vi "Main.vi"(8 "error in":errorcluster, 11 "TCP Server in":refnum<class "TCP Server.lvclass">) -> (0 "error out":errorcluster, 3 "TCP Server out":refnum<class "TCP Server.lvclass">)   [LabVIEW 2017, in "_TCP Server.lvlib" / "TCP Server.lvclass"]
doc: "The <b>Queued Message Handler</b> of the Worker that owns this VI."
uses:
  TCP Server.lvclass
  C:/SC/Source Code/VIPM/LabVIEW 20xx/vi.lib/addons/_Workers/Library/Classes/Worker/Worker.lvclass
  TCP Server.lvclass/TCP Server.ctl
  Initialization Data.ctl
  Response Cases.ctl
  <vilib>/addons/_Workers/Library/Case Label.ctl
  rql_Create Read Worker.ctl
  TCP Read/Initialization Data.ctl
  TCP Read/Response Cases.ctl
  <vilib>/addons/_Workers/Library/Classes/Message Queue/Message Queue.lvclass
  rqp_Start Listening.ctl
  TCP Listener/rqp_Listen for Connections.ctl
  rqp_Disconnect Clients.ctl
  rqp_Send String to Clients.ctl
  TCP Client Data.ctl
  <vilib>/addons/_Workers/Library/Classes/Message/Priority.ctl
  rsp_Connection Notify.ctl
  <vilib>/Utility/error.llb/Error Cluster From Error Code.vi
  <vilib>/addons/_Workers/Library/Classes/Worker/Worker.lvclass
  <vilib>/ErrorRing/Error Ring.xnode
  TCP Listener/TCP Listener.lvclass
  <vilib>/addons/_Workers/Library/Classes/Message/Message.lvclass
  TCP Read/TCP Read.lvclass
  <vilib>/addons/_Workers/Library/Workers.lvlib
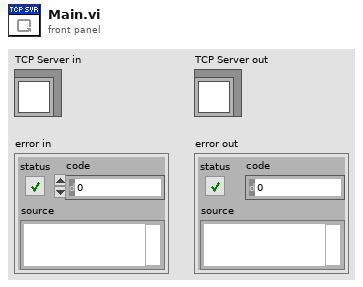
[diagram p1: front panel]
types:
  T1 = typedef "_TCP Server.lvlib/TCP Server.lvclass/Initialization Data.ctl" = cluster{"Response Cases":T2}
  T2 = typedef "_TCP Server.lvlib/TCP Server.lvclass/Response Cases.ctl" = cluster{"Incoming Data":T3, "Connection Notify":T3}
  T3 = typedef "Workers.lvlib/Case Label.ctl" = string
  T4 = typedef "_TCP Server.lvlib/TCP Read.lvclass/Initialization Data.ctl" = cluster{"Response Cases":T5, "Connection ID":refnum<k5>, "Forwarding Queue":refnum<class "Message Queue.lvclass">, "Forwarding Case":T3, "Client Name":string}
  T5 = typedef "_TCP Server.lvlib/TCP Read.lvclass/Response Cases.ctl" = cluster{"Connection Lost":T3}
  T6 = typedef "_TCP Server.lvlib/TCP Server.lvclass/rql_Create Read Worker.ctl" = cluster{"Connection ID":refnum<k5>, "Client Name":string}
  T7 = typedef "_TCP Server.lvlib/TCP Listener.lvclass/rqp_Listen for Connections.ctl" = cluster{"Server Name":string, "Server IP Address":u32, "Server Port":u16}
  T8 = typedef "_TCP Server.lvlib/TCP Server.lvclass/rqp_Start Listening.ctl" = cluster{"Server Name":string, "Server IP Address":string, "Server Port":u16}
  T9 = typedef "_TCP Server.lvlib/TCP Server.lvclass/rqp_Disconnect Clients.ctl" = cluster{"TCP Client Names":string[]}
  T10 = typedef "_TCP Server.lvlib/TCP Server.lvclass/rqp_Send String to Clients.ctl" = cluster{"TCP Client Names":string[], "String to Send":string}
  T11 = typedef "_TCP Server.lvlib/TCP Server.lvclass/rsp_Connection Notify.ctl" = cluster{"Client Name":string, "IP Address":string, "Connected?":bool}
  T12 = typedef "Workers.lvlib/Message.lvclass/Priority.ctl" = enum16{"Low", "Normal", "High"}
  T13 = typedef "_TCP Server.lvlib/TCP Server.lvclass/TCP Client Data.ctl" = cluster{"Connection ID":refnum<k5>, "Client Name":string, "IP Address":string}
  T14 = typedef "_TCP Server.lvlib/TCP Listener.lvclass/rsp_Add Listener.ctl" = cluster{"listener ID":refnum<k5>}
  T15 = typedef "_TCP Server.lvlib/TCP Listener.lvclass/rsp_New Connection.ctl" = cluster{"Connection ID":refnum<k5>, "Client Name":string, "IP Address":string}
  T16 = typedef "_TCP Server.lvlib/TCP Read.lvclass/rsp_Connection Lost.ctl" = cluster{"Connection ID":refnum<k5>, "TCP Read Queue":refnum<class "Message Queue.lvclass">}
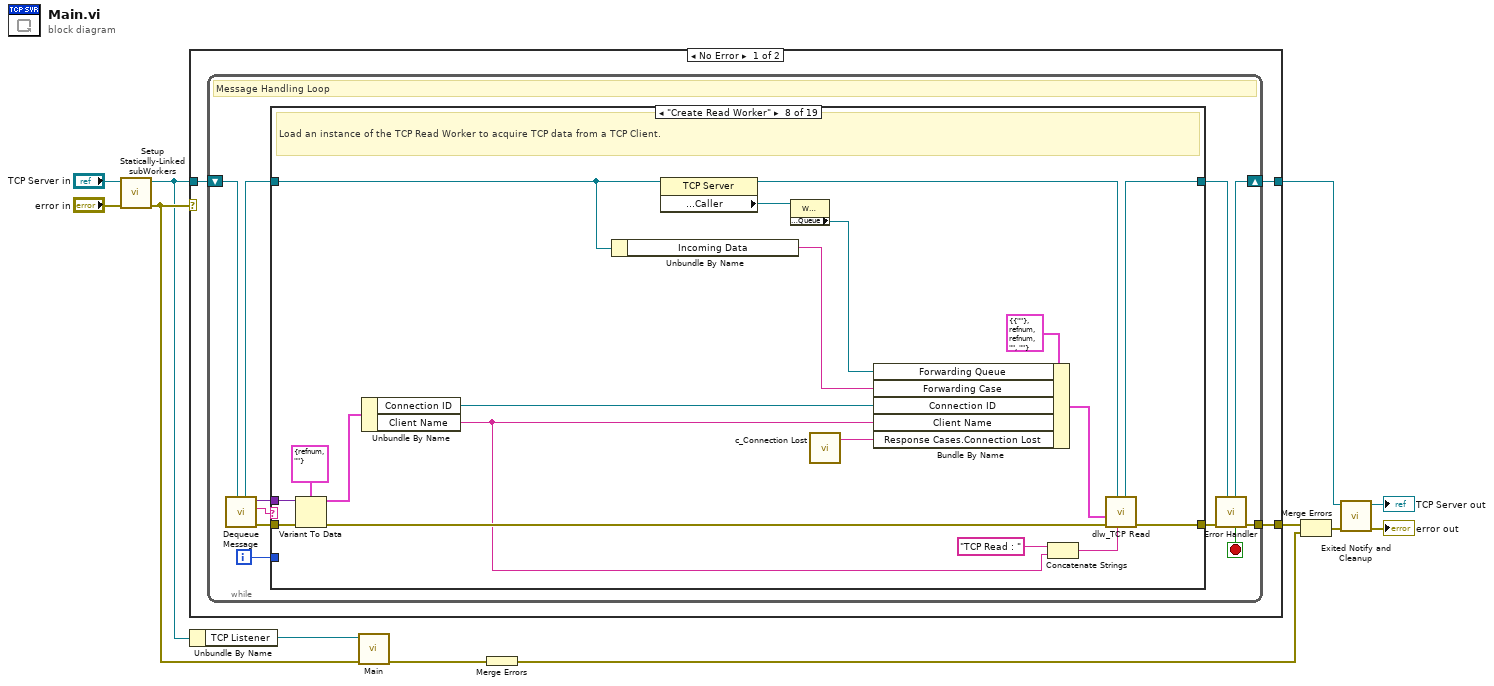
[diagram p0: block diagram]
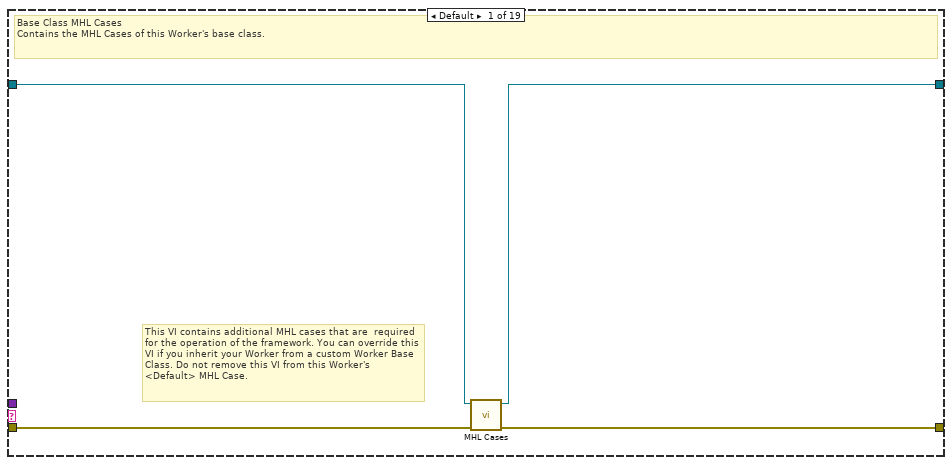
[diagram p2: hidden frame]
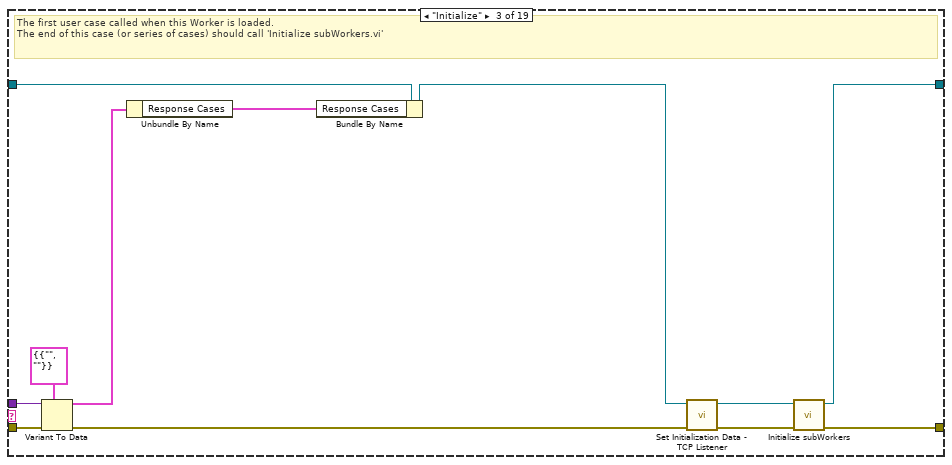
[diagram p4: hidden frame]
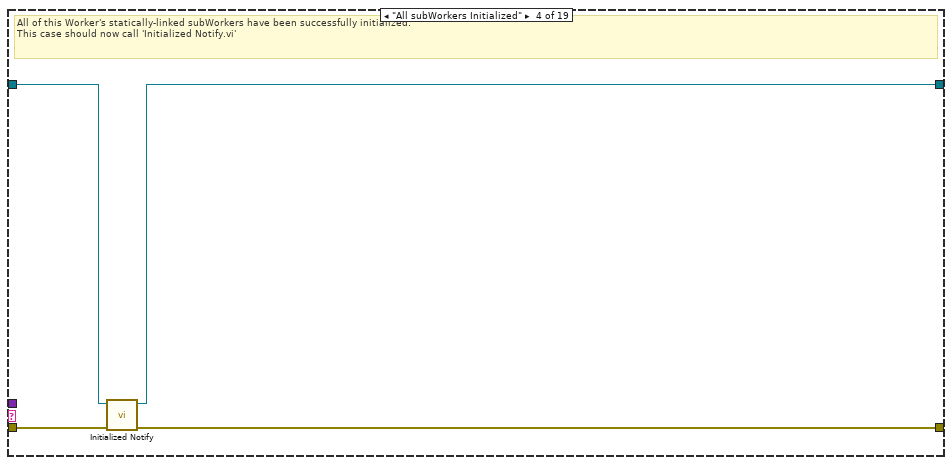
[diagram p5: hidden frame]
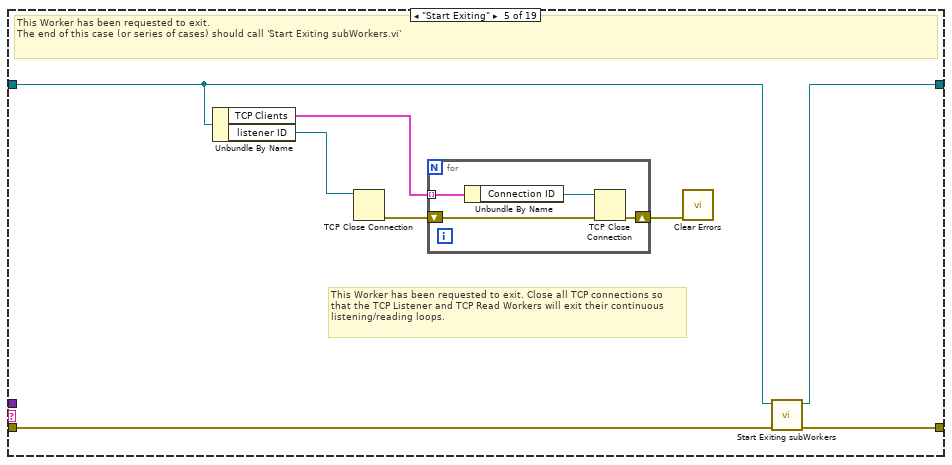
[diagram p6: hidden frame]
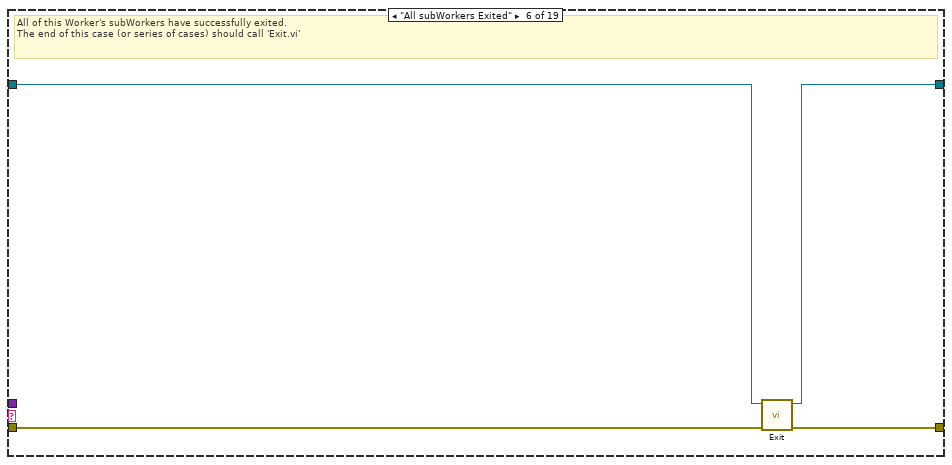
[diagram p7: hidden frame]
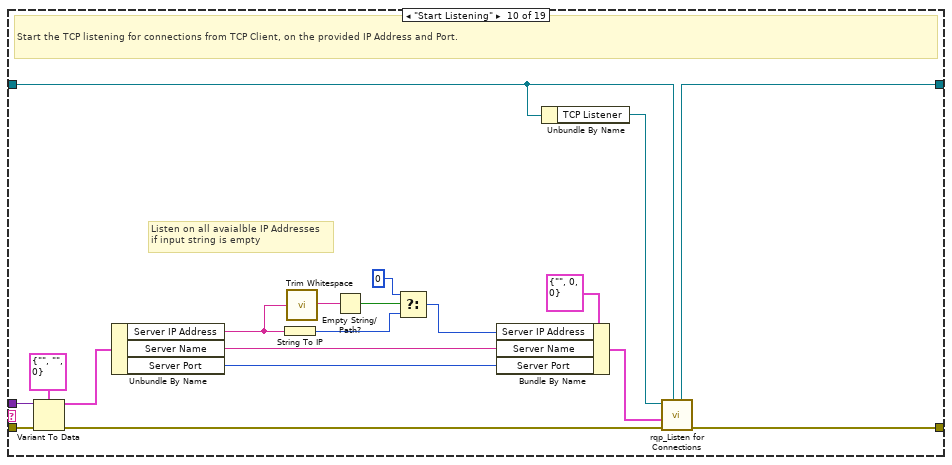
[diagram p10: hidden frame]
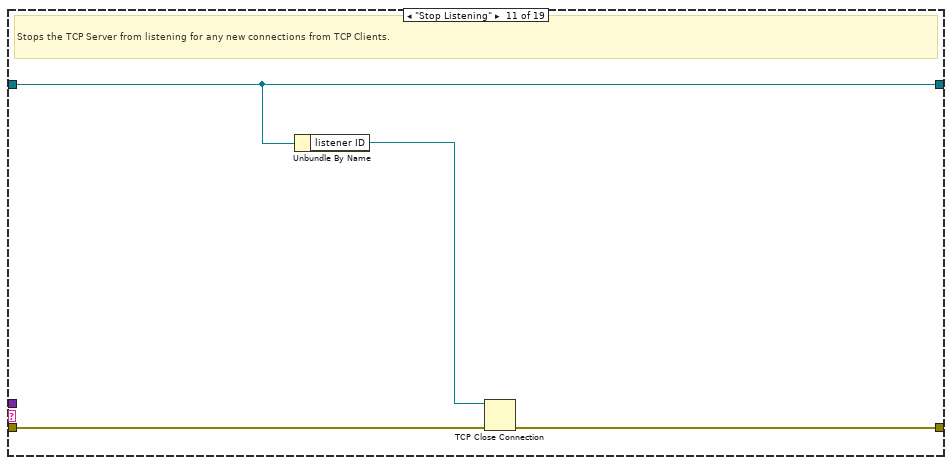
[diagram p11: hidden frame]
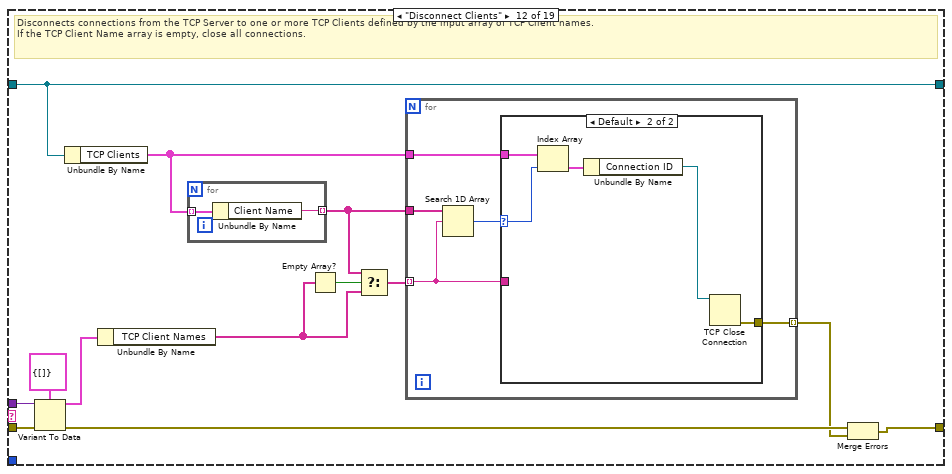
[diagram p12: hidden frame]
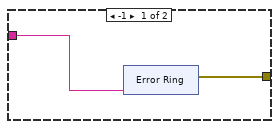
[diagram p13: hidden frame]
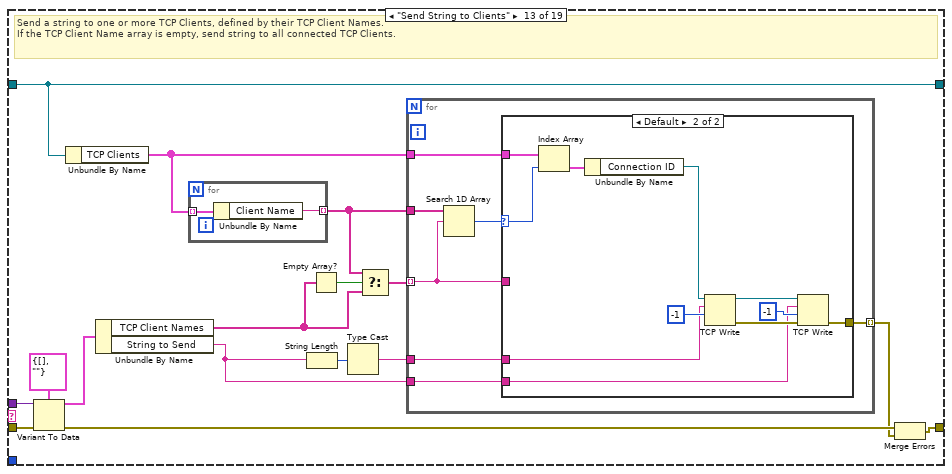
[diagram p14: hidden frame]
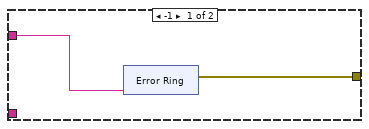
[diagram p15: hidden frame]
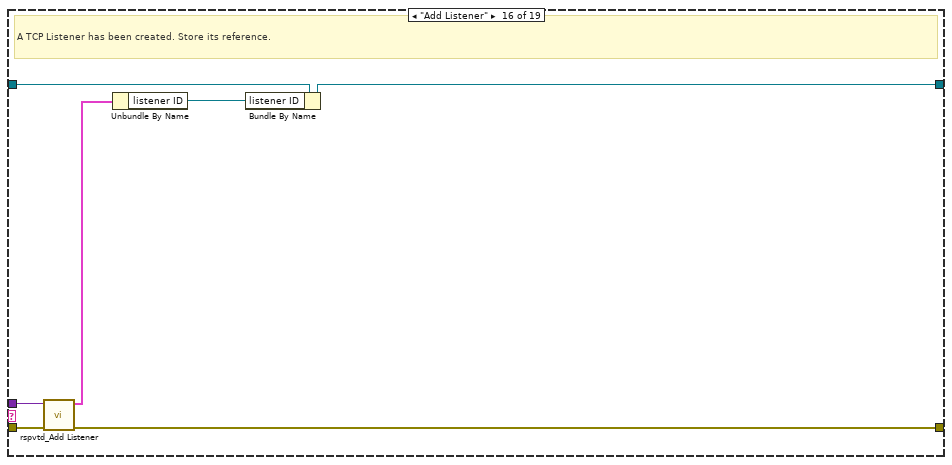
[diagram p18: hidden frame]
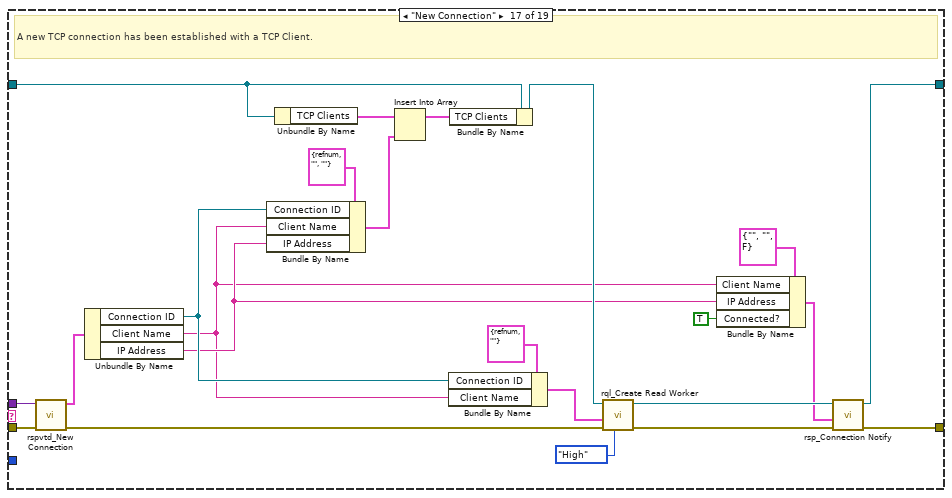
[diagram p19: hidden frame]
diagram:
  n1 = call "Setup Statically-Linked subWorkers.vi"("error in"="error in", "TCP Server in"="TCP Server in") -> ("error out"=w6:errorcluster, "TCP Server out"=w4:refnum<class "TCP Server.lvclass">)  [unwired: 8 in]
  n2 = case shown="No Error" w6 {
    tunnel: w4 -> [w13 w273]
    tunnel: [w15 w274] -> w11
    tunnel: [w14 w272] -> w12
    selector: w6 -> [_ w275]
    frame No Error {
      n3 = while {
        shift-right: [w24] -> w14
        shift-left: w13 -> [w26]
        tunnel: [w25] -> w15
        i -> [w17]
        stop <- w18 stop-if-true
        # "Message Handling Loop"
        n4 = call-dynamic "Dequeue Message.vi"("Worker"=w26) -> ("error out"=w23:errorcluster, "Case out"=w19:string, "Data out"=w16:variant, "Worker out"=w21:refnum<class "TCP Server.lvclass">)  [unwired: 6 in, 1 out]
        n5 = case "Worker MHL Case Structure (DO NOT CHANGE LABEL NAME)" shown="\"Create Read Worker\"" w19 {
          tunnel: w23 -> [w30 w31 w42 w48 w54 w64 w66 w85 w87 w106 w110 w123 w160 w191 w193 w200 w223 w225 w242]
          tunnel: [w29 w31 w44 w47 w56 w63 w66 w80 w87 w101 w109 w114 w149 w191 w193 w198 w208 w225 w235] -> w22
          tunnel: w21 -> [w28 w32 w41 w46 w53 w62 w65 w76 w86 w99 w108 w118 w153 w190 w192 w199 w218 w224 w238]
          tunnel: [w27 w32 w43 w45 w55 w61 w65 w79 w86 w100 w108 w118 w153 w190 w192 w195 w206 w224 w233] -> w20
          tunnel: w17 -> [_ _ _ _ _ _ _ _ _ _ _ _ _ _ _ _ _ _ _]
          tunnel: w16 -> [_ _ w39 _ _ _ _ w82 _ w104 _ w120 w157 _ _ w197 w222 _ w240]
          frame Default {
            # "This VI contains additional MHL cases that are  required for the operation of the framework. You can override this VI if you inherit your Worker from a custom Worker Base Class. Do not remove this VI from this Worker's <Default> MHL Case."
            # "Base Class MHL Cases\nContains the MHL Cases of this Worker's base class."
            n6 = call-dynamic "MHL Cases.vi"("error in"=w30, "Worker in"=w28) -> ("error out"=w29:errorcluster, "Worker out"=w27:refnum<class "TCP Server.lvclass">)  [unwired: 8 in]
          }
          frame "------------ FRAMEWORK CASES -----------" {
            # "Start of Workers Framework Cases"
          }
          frame "Initialize" {
            # "The first user case called when this Worker is loaded.\nThe end of this case (or series of cases) should call 'Initialize subWorkers.vi'"
            n7 = Variant To Data(error in=w42, type=T1 {"Response Cases"={"Incoming Data"="", "Connection Notify"=""}} ("Cluster"), Variant=w39) -> (data=w38:T1, error out=w40:errorcluster)
            n8 = Unbundle By Name(w38) -> ("Response Cases"=w37:T2)
            n9 = Bundle By Name(cluster=w41, "Response Cases"=w37) -> (w33:refnum<class "TCP Server.lvclass">)
            n10 = call "Set Initialization Data - TCP Listener.vi"("error in"=w40, "TCP Server in"=w33) -> ("error out"=w35:errorcluster, "TCP Server out"=w34:refnum<class "TCP Server.lvclass">)  [unwired: 8 in]
            n11 = call-dynamic "Initialize subWorkers.vi"("error in"=w35, "Worker"=w34) -> ("error out"=w44:errorcluster, "dup Worker out"=w43:refnum<class "TCP Server.lvclass">)  [unwired: 8 in]
          }
          frame "All subWorkers Initialized" {
            # "All of this Worker's statically-linked subWorkers have been successfully initialized.\nThis case should now call 'Initialized Notify.vi'"
            n12 = call-dynamic "Initialized Notify.vi"("error in"=w48, "Worker"=w46) -> ("error out"=w47:errorcluster, "dup Worker out"=w45:refnum<class "TCP Server.lvclass">)  [unwired: 8 in]
          }
          frame "Start Exiting" {
            # "This Worker has been requested to exit. Close all TCP connections so that the TCP Listener and TCP Read Workers will exit their continuous listening/reading loops."
            # "This Worker has been requested to exit. \nThe end of this case (or series of cases) should call 'Start Exiting subWorkers.vi'"
            n13 = Unbundle By Name(w53) -> ("TCP Clients"=w50:T13[], "listener ID"=w51:refnum<k5>)
            n14 = TCP Close Connection(connection ID=w51) -> (error out=w52:errorcluster)  [unwired: 2 in, 1 out]
            n15 = for {
              shift-right: [w59] -> w49
              shift-left: w52 -> [w60]
              tunnel: w50 -> [w58] mode=indexing
              n16 = Unbundle By Name(w58) -> ("Connection ID"=w57:refnum<k5>)
              n17 = TCP Close Connection(connection ID=w57, error in (no error)=w60) -> (error out=w59:errorcluster)  [unwired: 1 in, 1 out]
            }
            n18 = call <vilib>:"Clear Errors.vi"("error in (no error)"=w49) -> ()  [unwired: 5 in, 2 out]
            n19 = call-dynamic "Start Exiting subWorkers.vi"("error_in"=w54, "Worker"=w53) -> ("error out"=w56:errorcluster, "dup Worker out"=w55:refnum<class "TCP Server.lvclass">)  [unwired: 8 in]
          }
          frame "All subWorkers Exited" {
            # "All of this Worker's subWorkers have successfully exited. \nThe end of this case (or series of cases) should call 'Exit.vi'"
            n20 = call-dynamic "Exit.vi"("error_in"=w64, "Worker"=w62) -> ("error out"=w63:errorcluster, "dup Worker out"=w61:refnum<class "TCP Server.lvclass">)  [unwired: 8 in]
          }
          frame "------------- LOCAL API CASES -------------" {
            # "Start of Workers Local API Cases"
          }
          frame "Create Read Worker" {
            # "Load an instance of the TCP Read Worker to acquire TCP data from a TCP Client."
            n21 = Variant To Data(error in=w85, type=T6 {"Connection ID"=refnum, "Client Name"=""} ("Data"), Variant=w82) -> (data=w81:T6, error out=w84:errorcluster)
            n22 = Unbundle By Name(w81) -> ("Connection ID"=w72:refnum<k5>, "Client Name"=w70:string)
            n23 = Unbundle By Name(w76) -> ("Incoming Data"=w75:T3)
            n24 = property class="TCP Server"(reference=w76) -> (reference out=w74:refnum<class "TCP Server.lvclass">, "Accessors:Read:Public API:Caller"=w73:refnum<class "Worker.lvclass">)  [unwired: 1 in, 1 out]
            n25 = property class="Worker.lvclass"(reference=w73) -> ("Accessors:Read:Public API:Queue"=w67:refnum<class "Message Queue.lvclass">)  [unwired: 1 in, 2 out]
            n26 = call "c_Connection Lost.vi"() -> ("Case Label"=w68:T3)  [unwired: 1 in]
            n27 = Bundle By Name(cluster=T4 {"Response Cases"={"Connection Lost"=""}, "Connection ID"=refnum, "Forwarding Queue"=refnum, "Forwarding Case"="", "Client Name"=""} ("Initialization Data"), "Forwarding Queue"=w67, "Forwarding Case"=w75, "Connection ID"=w72, "Client Name"=w70, "Response Cases.Connection Lost"=w68) -> (w77:T4)
            n28 = Concatenate Strings("TCP Read : " ("Worker Alias"), w70) -> (w69:string)
            n29 = call "dlw_TCP Read.vi"("Worker Alias"=w69, "Caller in"=w74, "error in"=w84, "Initialization Data"=w77) -> ("error out"=w80:errorcluster, "dup Caller out"=w79:refnum<class "TCP Server.lvclass">)  [unwired: 5 in, 1 out]
          }
          frame "------------- PUBLIC API CASES -------------" {
            # "Start of Workers Public API Cases"
          }
          frame "Start Listening" {
            # "Listen on all avaialble IP Addresses\nif input string is empty"
            # "Start the TCP listening for connections from TCP Client, on the provided IP Address and Port."
            n30 = Variant To Data(error in=w106, type=T8 {"Server Name"="", "Server IP Address"="", "Server Port"=0} ("Data"), Variant=w104) -> (data=w103:T8, error out=w102:errorcluster)
            n31 = Unbundle By Name(w103) -> ("Server IP Address"=w90:string, "Server Name"=w91:string, "Server Port"=w92:u16)
            n32 = String To IP(1:w90) -> (0:w95:u32)
            n33 = call <vilib>:"Trim Whitespace.vi"("string"=w90) -> ("trimmed string"=w93:string)  [unwired: 1 in]
            n34 = Empty String/Path?(string/path=w93) -> (empty?=w94:bool)
            n35 = Select(t=u32 0, s=w94, f=w95) -> (s? t:f=w96:u32)
            n36 = Bundle By Name(cluster=T7 {"Server Name"="", "Server IP Address"=0, "Server Port"=0} ("Data in"), "Server IP Address"=w96, "Server Name"=w91, "Server Port"=w92) -> (w88:T7)
            n37 = Unbundle By Name(w99) -> ("TCP Listener"=w98:refnum<class "TCP Listener.lvclass">)
            n38 = call "rqp_Listen for Connections.vi"("Caller in"=w99, "error in"=w102, "Data in"=w88, "TCP Listener in"=w98) -> ("error out"=w101:errorcluster, "dup Caller out"=w100:refnum<class "TCP Server.lvclass">)  [unwired: 5 in, 1 out]
          }
          frame "Stop Listening" {
            # "Stops the TCP Server from listening for any new connections from TCP Clients."
            n39 = Unbundle By Name(w108) -> ("listener ID"=w107:refnum<k5>)
            n40 = TCP Close Connection(connection ID=w107, error in (no error)=w110) -> (error out=w109:errorcluster)  [unwired: 1 in, 1 out]
          }
          frame "Disconnect Clients" {
            # "Disconnects connections from the TCP Server to one or more TCP Clients defined by the input array of TCP Client names.\nIf the TCP Client Name array is empty, close all connections."
            n41 = Variant To Data(error in=w123, type=T9 {"TCP Client Names"=[]} ("Data"), Variant=w120) -> (data=w119:T9, error out=w122:errorcluster)
            n42 = Unbundle By Name(w118) -> ("TCP Clients"=w115:T13[])
            n43 = Unbundle By Name(w119) -> ("TCP Client Names"=w116:string[])
            n44 = for {
              tunnel: w115 -> [w125] mode=indexing
              tunnel: [w124] -> w112 mode=indexing
              n45 = Unbundle By Name(w125) -> ("Client Name"=w124:string)
            }
            n46 = Empty Array?(array=w116) -> (empty?=w117:bool)
            n47 = Select(t=w112, s=w117, f=w116) -> (s? t:f=w111:string[])
            n48 = for {
              tunnel: w111 -> [w127] mode=indexing
              tunnel: w112 -> [w130]
              tunnel: w115 -> [w129]
              tunnel: [w126] -> w113 mode=indexing
              n49 = Search 1D Array(1D array=w130, element=w127) -> (index of element=w128:i32)  [unwired: 1 in]
              n50 = case shown="Default" w128 {
                selector: w128 -> [_ w143]
                tunnel: w129 -> [_ w144]
                tunnel: w127 -> [w132 _]
                tunnel: [w131 w140] -> w126
                frame -1 {
                  n51 = xnode "Error Ring"("parameter 0"=w132) -> ("error out"=w131:errorcluster)
                }
                frame Default {
                  n52 = Index Array(array=w144, index=w143) -> (element=w142:T13)
                  n53 = Unbundle By Name(w142) -> ("Connection ID"=w141:refnum<k5>)
                  n54 = TCP Close Connection(connection ID=w141) -> (error out=w140:errorcluster)  [unwired: 2 in, 1 out]
                }
              }
            }
            n55 = Merge Errors(w122, w113) -> (w114:errorcluster)
          }
          frame "Send String to Clients" {
            # "Send a string to one or more TCP Clients, defined by their TCP Client Names.\nIf the TCP Client Name array is empty, send string to all connected TCP Clients."
            n56 = Variant To Data(error in=w160, type=T10 {"TCP Client Names"=[], "String to Send"=""} ("Data"), Variant=w157) -> (data=w152:T10, error out=w159:errorcluster)
            n57 = Unbundle By Name(w153) -> ("TCP Clients"=w154:T13[])
            n58 = Unbundle By Name(w152) -> ("TCP Client Names"=w155:string[], "String to Send"=w147:string)
            n59 = for {
              tunnel: w154 -> [w162] mode=indexing
              tunnel: [w161] -> w145 mode=indexing
              n60 = Unbundle By Name(w162) -> ("Client Name"=w161:string)
            }
            n61 = String Length(string=w147) -> (length=w151:i32)
            n62 = Empty Array?(array=w155) -> (empty?=w156:bool)
            n63 = Type Cast(x=w151) -> (*(type *) &x=w150:string)  [unwired: 1 in]
            n64 = Select(t=w145, s=w156, f=w155) -> (s? t:f=w146:string[])
            n65 = for {
              tunnel: w146 -> [w166] mode=indexing
              tunnel: w145 -> [w169]
              tunnel: w154 -> [w168]
              tunnel: [w165] -> w148 mode=indexing
              tunnel: w150 -> [w164]
              tunnel: w147 -> [w163]
              n66 = Search 1D Array(1D array=w169, element=w166) -> (index of element=w167:i32)  [unwired: 1 in]
              n67 = case shown="Default" w167 {
                selector: w167 -> [_ w188]
                tunnel: w168 -> [_ w189]
                tunnel: w166 -> [w171 _]
                tunnel: [w170 w181] -> w165
                tunnel: w164 -> [_ w180]
                tunnel: w163 -> [_ w179]
                frame -1 {
                  n68 = xnode "Error Ring"("parameter 0"=w171) -> ("error out"=w170:errorcluster)
                }
                frame Default {
                  n69 = Index Array(array=w189, index=w188) -> (element=w187:T13)
                  n70 = Unbundle By Name(w187) -> ("Connection ID"=w182:refnum<k5>)
                  n71 = TCP Write(connection ID=w182, data in=w180, 9:-1 ("timeout ms (25000)")) -> (connection ID out=w184:refnum<k5>, error out=w183:errorcluster)  [unwired: 1 in, 1 out]
                  n72 = TCP Write(connection ID=w184, data in=w179, error in (no error)=w183, 9:-1 ("timeout ms (25000)")) -> (error out=w181:errorcluster)  [unwired: 2 out]
                }
              }
            }
            n73 = Merge Errors(w159, w148) -> (w149:errorcluster)
          }
          frame "------------- RESPONSE CASES --------------" {
            # "Start of Workers Response Cases"
          }
          frame "~~~~~~~~~~ TCP Listener ~~~~~~~~~~ " {
          }
          frame "Add Listener" {
            # "A TCP Listener has been created. Store its reference."
            n74 = call "rspvtd_Add Listener.vi"("error in"=w200, "Data in"=w197) -> ("error out"=w198:errorcluster, "Data out"=w196:T14)  [unwired: 8 in]
            n75 = Unbundle By Name(w196) -> ("listener ID"=w194:refnum<k5>)
            n76 = Bundle By Name(cluster=w199, "listener ID"=w194) -> (w195:refnum<class "TCP Server.lvclass">)
          }
          frame "New Connection" {
            # "A new TCP connection has been established with a TCP Client."
            n77 = call "rspvtd_New Connection.vi"("error in"=w223, "Data in"=w222) -> ("error out"=w215:errorcluster, "Data out"=w221:T15)  [unwired: 8 in]
            n78 = Unbundle By Name(w221) -> ("Connection ID"=w210:refnum<k5>, "Client Name"=w201:string, "IP Address"=w202:string)
            n79 = Bundle By Name(cluster=T13 {"Connection ID"=refnum, "Client Name"="", "IP Address"=""} ("new element/subarray"), "Connection ID"=w210, "Client Name"=w201, "IP Address"=w202) -> (w216:T13)
            n80 = Unbundle By Name(w218) -> ("TCP Clients"=w220:T13[])
            n81 = Insert Into Array(array=w220, new element=w216) -> (w219:T13[])  [unwired: 1 in]
            n82 = Bundle By Name(cluster=T6 {"Connection ID"=refnum, "Client Name"=""} ("Data in"), "Connection ID"=w210, "Client Name"=w201) -> (w211:T6)
            n83 = Bundle By Name(cluster=w218, "TCP Clients"=w219) -> (w213:refnum<class "TCP Server.lvclass">)
            n84 = call "rql_Create Read Worker.vi"("Message Priority"=Priority."High", "error in"=w215, "Data in"=w211, "TCP Server in"=w213) -> ("error out"=w214:errorcluster, "dup TCP Server out"=w207:refnum<class "TCP Server.lvclass">)  [unwired: 6 in]
            n85 = Bundle By Name(cluster=T11 {"Client Name"="", "IP Address"="", "Connected?"=FALSE} ("Data in"), "Client Name"=w201, "IP Address"=w202, "Connected?"=TRUE) -> (w204:T11)
            n86 = call "rsp_Connection Notify.vi"("error in"=w214, "Data in"=w204, "TCP Server in"=w207) -> ("error out"=w208:errorcluster, "dup TCP Server out"=w206:refnum<class "TCP Server.lvclass">)  [unwired: 7 in]
          }
          frame "~~~~~~~~~~ TCP Read ~~~~~~~~~~~~ " {
          }
          frame "Connection Lost" {
            # "Needed in case the TCP connection is cut from the TCP Client side"
            # "A connection to a TCP Client has been lost. Notify the Caller."
            n87 = call "rspvtd_Connection Lost.vi"("error in"=w242, "Data in"=w240) -> ("error out"=w241:errorcluster, "Data out"=w237:T16)  [unwired: 8 in]
            n88 = Unbundle By Name(w237) -> ("Connection ID"=w226:refnum<k5>, "TCP Read Queue"=w236:refnum<class "Message Queue.lvclass">)
            n89 = call-dynamic "Worker Start Exiting.vi"("error_in"=w241, "Message Queue"=w236, "Worker"=w238) -> ("error out"=w239:errorcluster, "dup Worker out"=w234:refnum<class "TCP Server.lvclass">)  [unwired: 7 in]
            n90 = Unbundle By Name(w234) -> ("TCP Clients"=w230:T13[])
            n91 = TCP Close Connection(connection ID=w226) -> (error out=w227:errorcluster)  [unwired: 2 in, 1 out]
            n92 = call <vilib>:"Clear Errors.vi"("error in (no error)"=w227) -> ()  [unwired: 5 in, 2 out]
            n93 = for {
              tunnel: w230 -> [w271] mode=indexing
              tunnel: [w270] -> w231
              tunnel: [w269] -> w228
              tunnel: [w268] -> w232
              tunnel: [w267] -> w229
              tunnel: w226 -> [w265]
              i -> [w270]
              stop <- w268 stop-if-true
              n94 = Unbundle By Name(w271) -> ("IP Address"=w267:string, "Client Name"=w269:string, "Connection ID"=w266:refnum<k5>)
              n95 = Equal?(x=w266, y=w265) -> (x = y?=w268:bool)
            }
            n96 = case shown="True" w232 {
              tunnel: w239 -> [w244 w264]
              tunnel: [w243 w263] -> w235
              tunnel: w234 -> [w246 w262]
              tunnel: [w246 w261] -> w233
              tunnel: w231 -> [_ w260]
              tunnel: w230 -> [_ w259]
              tunnel: w229 -> [_ w254]
              tunnel: w228 -> [_ w253]
              frame False {
                n97 = xnode "Error Ring"() -> ("error out"=w245:errorcluster)
                n98 = Merge Errors(w244, w245) -> (w243:errorcluster)
              }
              frame True {
                n99 = Delete From Array(array=w259, index=w260) -> (array with subset deleted=w257:T13[])  [unwired: 1 in, 1 out]
                n100 = Bundle By Name(cluster=T11 {"Client Name"="", "IP Address"="", "Connected?"=FALSE} ("Data in"), "IP Address"=w254, "Client Name"=w253, "Connected?"=FALSE) -> (w255:T11)
                n101 = Bundle By Name(cluster=w262, "TCP Clients"=w257) -> (w258:refnum<class "TCP Server.lvclass">)
                n102 = call "rsp_Connection Notify.vi"("error in"=w264, "Data in"=w255, "TCP Server in"=w258) -> ("error out"=w263:errorcluster, "dup TCP Server out"=w261:refnum<class "TCP Server.lvclass">)  [unwired: 7 in]
              }
            }
          }
        }
        n103 = call-dynamic "Error Handler.vi"("Worker"=w20, "error_in"=w22) -> ("error out"=w25:errorcluster, "Stop Loop"=w18:bool, "Worker out"=w24:refnum<class "TCP Server.lvclass">)  [unwired: 7 in]
      }
    }
    frame Error {
      n104 = call-dynamic "Error Handler.vi"("Worker"=w273, "error_in"=w275) -> ("error out"=w274:errorcluster, "Worker out"=w272:refnum<class "TCP Server.lvclass">)  [unwired: 7 in, 1 out]
    }
  }
  n105 = Unbundle By Name(w4) -> ("TCP Listener"=w1:refnum<class "TCP Listener.lvclass">)
  n106 = call-dynamic "Main.vi"("error in"=w6, "TCP Listener in"=w1) -> ("error out"=w3:errorcluster)  [unwired: 8 in, 1 out]
  n107 = Merge Errors(w3) -> (w2:errorcluster)
  n108 = Merge Errors(w11, w2) -> (w8:errorcluster)
  n109 = call-dynamic "Exited Notify and Cleanup.vi"("error_in"=w8, "Worker"=w12) -> ("error out"=→"error out":errorcluster, "dup Worker out"=→"TCP Server out":refnum<class "TCP Server.lvclass">)  [unwired: 8 in]
